vi "bundled_error_handler.vi"(10 "session bundle in":T1={"relay session out"={"VISA resource out"="COM12", "error out"={"status"=FALSE, "code"=0, "source"=""}}, "kloehn session out"={"VISA resource out"="COM12", "error out"={"status"=FALSE, "code"=0, "source"=""}}, "LiCor session out"={"VISA resource out"="COM12", "error out"={"status"=FALSE, "code"=0, "source"=""}}}) -> (0 "LiCor error out":errorcluster, 1 "kloehn error out":errorcluster, 2 "relay error out":errorcluster, 3 "session bundle out":T1={"relay session out"={"VISA resource out"="COM12", "error out"={"status"=FALSE, "code"=0, "source"=""}}, "kloehn session out"={"VISA resource out"="COM12", "error out"={"status"=FALSE, "code"=0, "source"=""}}, "LiCor session out"={"VISA resource out"="COM12", "error out"={"status"=FALSE, "code"=0, "source"=""}}})   [LabVIEW 2010]
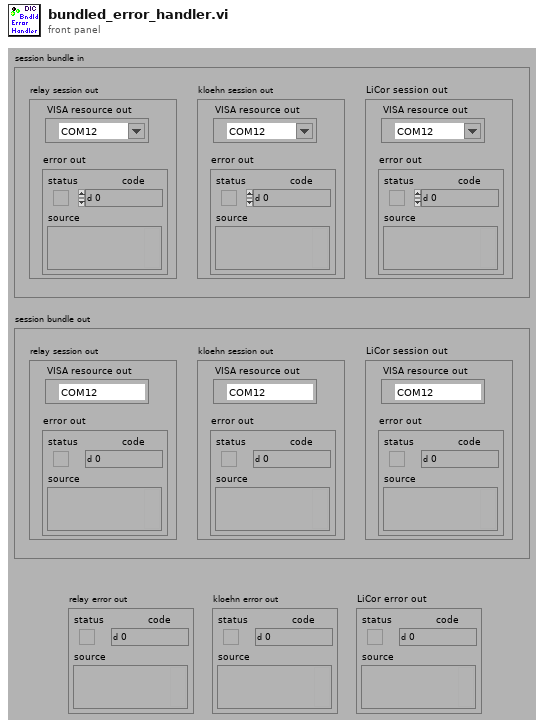
[diagram p1: front panel]
types:
  T1 = cluster{"relay session out":cluster{"VISA resource out":refnum<visa-resource-name>, "error out":errorcluster}, "kloehn session out":cluster{"VISA resource out":refnum<visa-resource-name>, "error out":errorcluster}, "LiCor session out":cluster{"VISA resource out":refnum<visa-resource-name>, "error out":errorcluster}}
  T2 = cluster{"VISA resource out":refnum<visa-resource-name>, "error out":errorcluster}
  T3 = cluster{"session out":cluster{"VISA resource out":refnum<visa-resource-name>, "error out":errorcluster}, "session out":cluster{"VISA resource out":refnum<visa-resource-name>, "error out":errorcluster}, "session out":cluster{"VISA resource out":refnum<visa-resource-name>, "error out":errorcluster}}
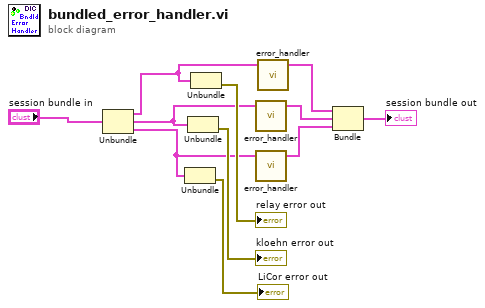
[diagram p0: block diagram]
diagram:
  n1 = Unbundle("session bundle in") -> ("relay session out"=w3:T2, "kloehn session out"=w2:T2, "LiCor session out"=w1:T2)
  n2 = Unbundle(w1) -> ("error out"=→"LiCor error out":errorcluster)  [unwired: 1 out]
  n3 = Unbundle(w2) -> ("error out"=→"kloehn error out":errorcluster)  [unwired: 1 out]
  n4 = Unbundle(w3) -> ("error out"=→"relay error out":errorcluster)  [unwired: 1 out]
  n5 = call "error_handler.vi"("session in"=w2) -> ("session out"=w10:T2)  [unwired: 2 in, 2 out]
  n6 = call "error_handler.vi"("session in"=w1) -> ("session out"=w9:T2)  [unwired: 2 in, 2 out]
  n7 = call "error_handler.vi"("session in"=w3) -> ("session out"=w11:T2)  [unwired: 2 in, 2 out]
  n8 = Bundle("session out"=w11, "session out"=w10, "session out"=w9) -> (→"session bundle out":T3)  [unwired: 1 in]
